vi "GT 2D Compare Set Prm.vi"(8 "error in (no error)":errorcluster caption="错误输入（无错误）", 9 "pPrm":T1, 10 "chn":i16, 11 "cardNum":i16) -> (0 "error out":errorcluster caption="错误输出", 1 "pPrm out":T1, 3 "function return":i16)   [LabVIEW 2020, in "gts.lvlib"]
doc: "GT_API GT_2DCompareSetPrm(short cardNum,short chn,T2DComparePrm *pPrm);"
uses:
  gts.lvlib
  dll/32bit/multi_card/gts.dll
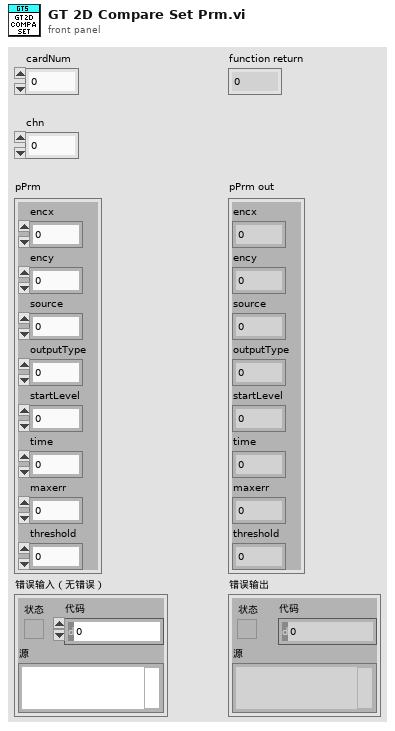
[diagram p1: front panel]
types:
  T1 = cluster{"encx":i16, "ency":i16, "source":i16, "outputType":i16, "startLevel":i16, "time":i16, "maxerr":i16, "threshold":i16}
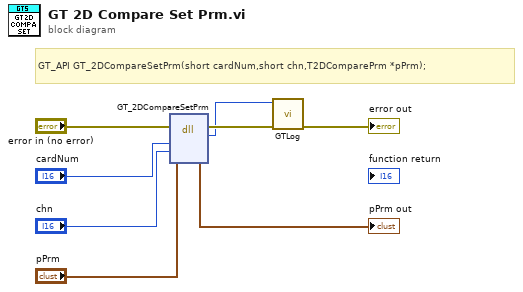
[diagram p0: block diagram]
diagram:
  # "GT_API GT_2DCompareSetPrm(short cardNum,short chn,T2DComparePrm *pPrm);"
  n1 = dll-call lib="C:/1228/dll/32bit/multi_card/gts.dll" fn="GT_2DCompareSetPrm"(error in="error in (no error)", "cardNum"="cardNum", "chn"="chn", "pPrm"="pPrm") -> (error out=w3:errorcluster, "返回类型"=w1:i16, "pPrm"=→"pPrm out":T1)  [unwired: 4 in, 1 out]
  n2 = call "GTLog.vi"("error in (no error)"=w3, "Numeric"=w1) -> ("error out"=→"error out":errorcluster)  [unwired: 9 in]
